vi "Rename File(冲突时的文件备份2013-03-27 14-07-26).vi"(8 "error in (no error)":errorcluster caption="错误输入（无错误）", 9 "NewFileName":path, 10 "SourceFileName":path, 11 "FileSystem 输入":refnum<class "FileSystem.lvclass"> caption="DNL_LabVIEW Object in") -> (0 "error out":errorcluster caption="错误输出", 3 "FileSystem 输出":refnum<class "FileSystem.lvclass"> caption="DNL_LabVIEW Object out")   [LabVIEW 2012, in "FileSystem.lvclass"]
uses:
  FileSystem.lvclass
  FileSystem.lvclass/FileSystem.ctl
  Microsoft.VisualBasic
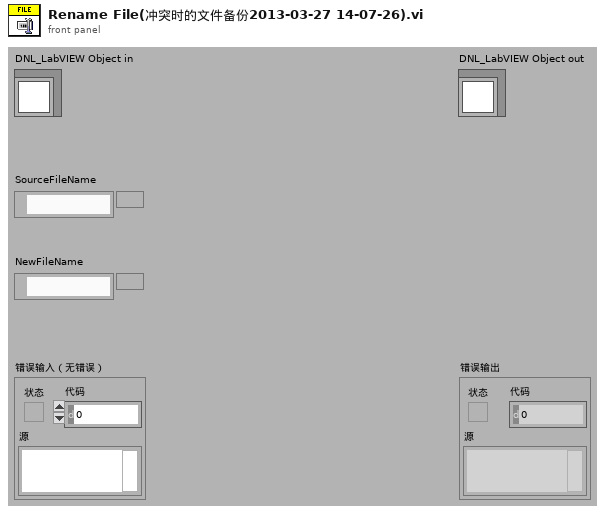
[diagram p1: front panel]
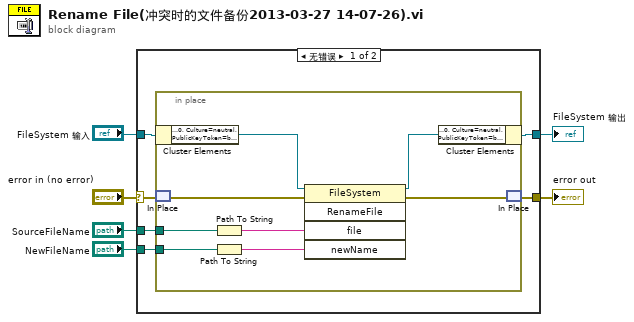
[diagram p0: block diagram]
diagram:
  n1 = case shown="无错误" "error in (no error)" {
    selector: "error in (no error)" -> [w11 w22]
    tunnel: [w10 w22] -> w5
    tunnel: [w7 w21] -> w3
    tunnel: "FileSystem 输入" -> [w12 w21]
    tunnel: "SourceFileName" -> [w9 _]
    tunnel: "NewFileName" -> [w8 _]
    frame No Error {
      n2 = in-place {
        in-place-border: w9 -> [w16]
        in-place-border: w8 -> [w14]
        n3 = in-place-cluster #1(w12) -> ("FileSystem"=w20:refnum<k24>)
        n4 = in-place-match #2(w11) -> (w18:errorcluster)
        n5 = Path To String(path=w16) -> (string=w15:string)
        n6 = Path To String(path=w14) -> (string=w13:string)
        n7 = invoke class="FileSystem" method="RenameFile"(reference=w20, error in=w18, "file"=w15, "newName"=w13) -> (reference out=w19:refnum<k24>, error out=w17:errorcluster)  [unwired: 1 in, 3 out]
        n8 = in-place-cluster #1("FileSystem"=w19) -> (w7:refnum<class "FileSystem.lvclass">)
        n9 = in-place-match #2(w17) -> (w10:errorcluster)
      }
    }
    frame Error {
    }
  }
  "error out" <- w5
  "FileSystem 输出" <- w3
